vi "BRA.vi"(0 "System no.":i32=1 min=1 max=4 step=1, 2 "Axes to command":string[](array[string]), 3 "Brake on":bool[](array[boolean]), 5 "error in":errorcluster) -> (19 "error out":errorcluster)   [LabVIEW 2020]
doc: "Switches brake for given axes on or off."
panel:
  # "Switches brake for given axes on or off."
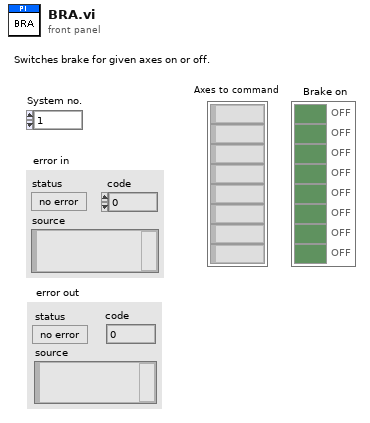
[diagram p1: front panel]
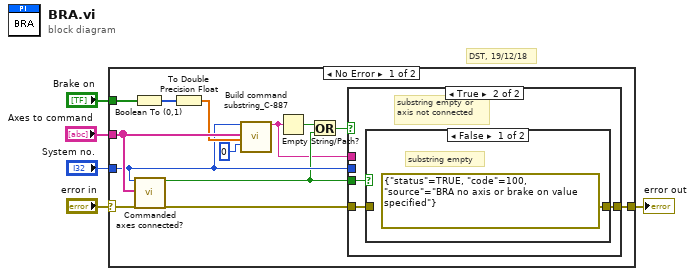
[diagram p0: block diagram]
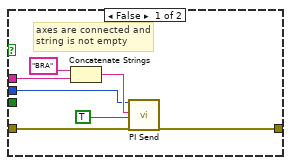
[diagram p2: hidden frame]
diagram:
  # "DST, 19/12/18"
  n1 = case shown="No Error" "error in" {
    selector: "error in" -> [w9 w31]
    tunnel: [w18 w31] -> w5
    tunnel: "System no." -> [w10 _]
    tunnel: "Axes to command" -> [w16 _]
    tunnel: "Brake on" -> [w14 _]
    frame No Error {
      n2 = Boolean To (0,1)(Boolean=w14) -> (0, 1=w13:i16[])
      n3 = call "Commanded axes connected?.vi"("System no."=w10, "Commanded axes"=w16, "error in"=w9) -> ("Controller error"=w8:bool, "error out"=w17:errorcluster)  [unwired: 1 in, 14 out]
      n4 = To Double Precision Float(number=w13) -> (double precision float=w11:dbl[])
      n5 = call "Build command substring_C-887.vi"("System no."=w10, "Affected axes"=w16, "Parameters"=w11, "No. of digits"=i16 0 ("No.of digits")) -> ("Command substring"=w6:string)  [unwired: 3 in, 12 out]
      n6 = Empty String/Path?(string/path=w6) -> (empty?=w7:bool)
      n7 = Or(x=w7, y=w8) -> (x .or. y?=w15:bool)
      n8 = case shown="True" w15 {
        tunnel: w6 -> [w24 _]
        tunnel: [w20 w28] -> w18
        tunnel: w17 -> [w21 w26]
        tunnel: w8 -> [_ w27]
        tunnel: w10 -> [w19 _]
        frame False {
          # "axes are connected and\nstring is not empty"
          n9 = Concatenate Strings("BRA", w24) -> (w22:string)
          n10 = call "PI Send.vi"("System no."=w19, "String to send"=w22, "Attach termination char.?"=TRUE ("Attach Linefeed?"), "error in"=w21) -> ("error out"=w20:errorcluster)  [unwired: 2 in, 13 out]
        }
        frame True {
          # "substring empty or \naxis not connected"
          n11 = case shown="False" w27 {
            tunnel: [errorcluster {"status"=TRUE, "code"=100, "source"="BRA no axis or brake on value specified"} ("error out") w30] -> w28
            tunnel: w26 -> [_ w30]
            frame False {
              # "substring empty"
            }
            frame True {
              # "commanded axis\nnot connected"
            }
          }
        }
      }
    }
    frame Error {
    }
  }
  "error out" <- w5
